vi "Init from Ref.vi"(8 "error in":errorcluster, 10 "MouseEventArgs":refnum<k24>, 11 "MouseEventArgs in":refnum<class "MouseEventArgs.lvclass">) -> (0 "error out":errorcluster, 3 "MouseEventArgs out":refnum<class "MouseEventArgs.lvclass">)   [LabVIEW 2024, in "SourceGrid.lvlib" / "MouseEventArgs.lvclass"]
uses:
  MouseEventArgs.lvclass
  MouseEventArgs.lvclass/MouseEventArgs.ctl
  System.Windows.Forms
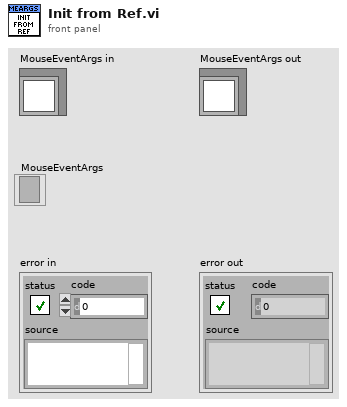
[diagram p1: front panel]
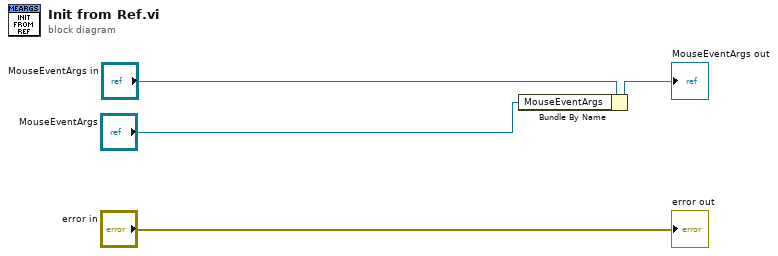
[diagram p0: block diagram]
diagram:
  n1 = Bundle By Name(cluster="MouseEventArgs in", "MouseEventArgs"="MouseEventArgs") -> (→"MouseEventArgs out":refnum<class "MouseEventArgs.lvclass">)
  "error out" <- "error in"
